vi "mro reset Command Stock(incomplete).vi"(8 "error in (no error)":errorcluster, 11 "status":i32) -> (0 "error out":errorcluster, 2 "function return":i8, 3 "status out":i32)   [LabVIEW 2016, in "mirao52e_32bit.lvlib"]
doc: "MIRAOEXPORT MroBoolean MIRAOCALL mro_resetCommandStock(\n int* status\n );"
uses:
  mirao52e_32bit.lvlib
  mirao52e.dll
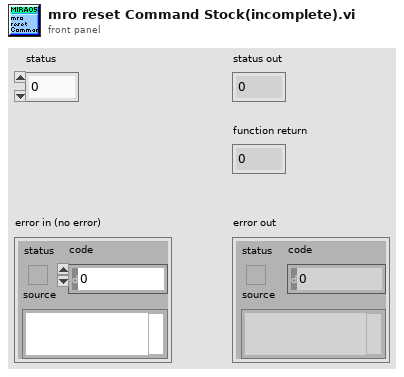
[diagram p1: front panel]
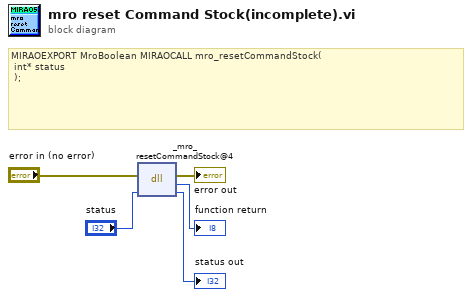
[diagram p0: block diagram]
diagram:
  # "MIRAOEXPORT MroBoolean MIRAOCALL mro_resetCommandStock(\n\tint* status\n\t);"
  n1 = dll-call lib="C:/Users/nvladim/Documents/Nikita-MDC/code/LabView/miraoDriver_32bit/mirao52e.*" fn="_mro_resetCommandStock@4"(error in="error in (no error)", "status"="status") -> (error out=→"error out":errorcluster, →"function return":i8, "status"=→"status out":i32)  [unwired: 2 in, 1 out]
